vi "MTest.vi"() -> ()   [LabVIEW 2017]
panel:
  in  "Clear W":bool
  out "error out 2":errorcluster
  out "read":string
  in  "Send Cmd":bool
  in  "sendStr":string
  out "RS-232":bool
  in  "Disconnect Com":bool
  in  "Connect Com":bool
  out "TesterVersion":string
  out "error out":errorcluster
  in  "9":bool
  in  "8":bool
  in  "7":bool
  in  "6":bool
  in  "1":bool
  in  "5":bool
  in  "4":bool
  in  "3":bool
  in  "2":bool
  out "DAQ":bool
  in  "Disconnect DAQ":bool
  in  "Connect DAQ":bool
  in  "Stop Button":bool
  in  "Remote":bool
  in  "UP":bool
  in  "DOWN":bool
  in  "V En":bool
  in  "FW":bool
  # "REDLER TECHNOLOGIES LTD"
  # "M Kinetics Tester"
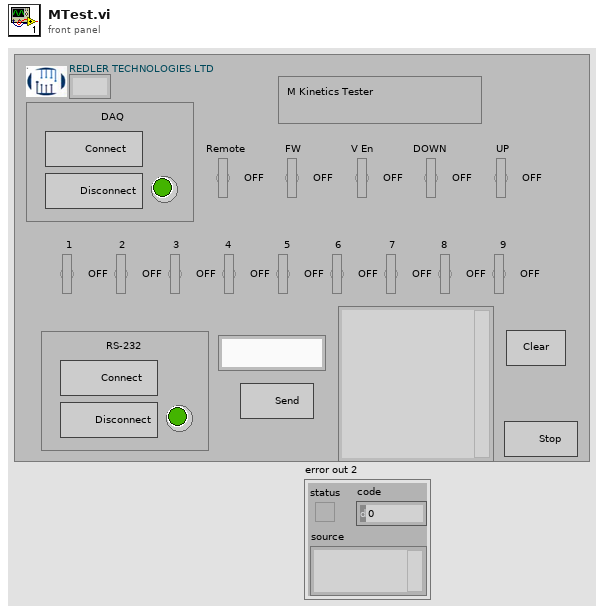
[diagram p1: front panel]
types:
  T1 = enum16{"Init", "0 ohm", "6 ohm", "13.2 ohm", "15 ohm", "25.9 ohm", "33 ohm", "Down", "Up", "Venable", "Firmware", "PowerSuply"}
  T2 = enum16{"Init", "0 ohm", "6 ohm", "13.2 ohm", "15 ohm", "25.9 ohm", "33 ohm", "Down", "Up", "Venable", "Firmware", "PowerSuply"}[]
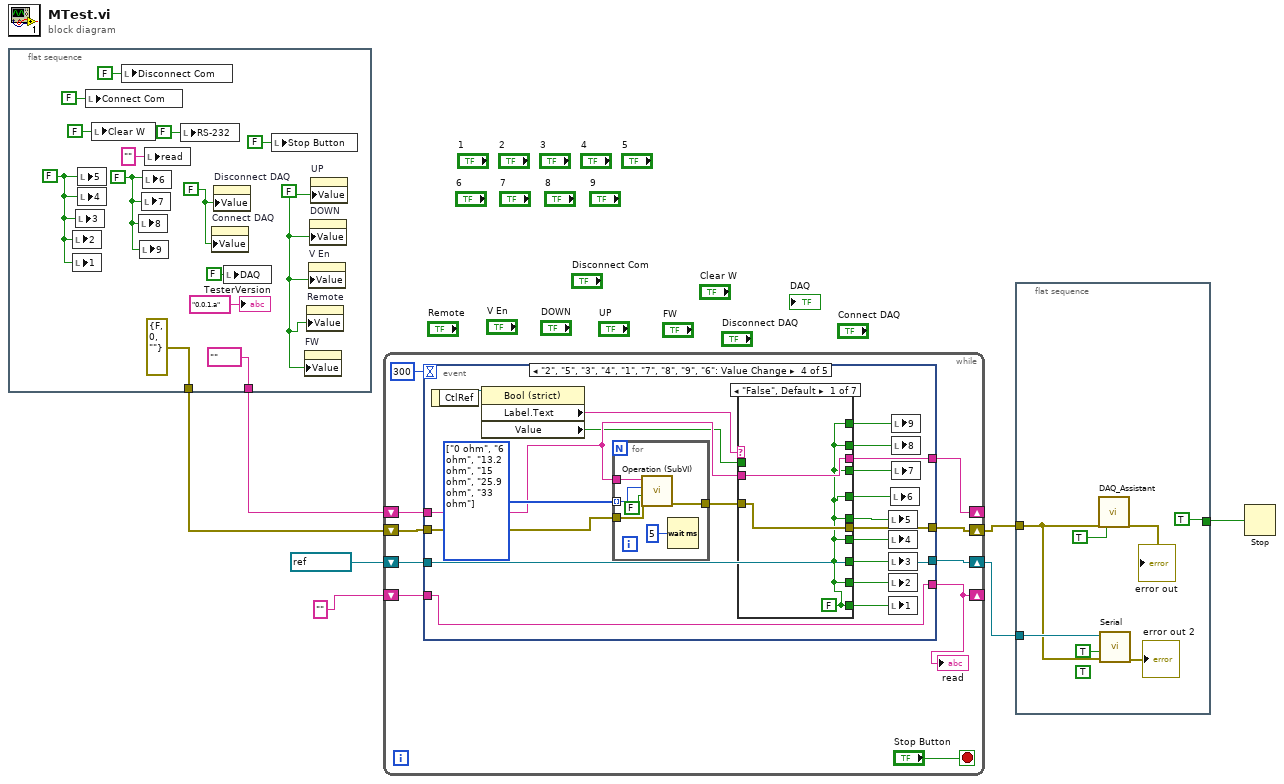
[diagram p0: block diagram]
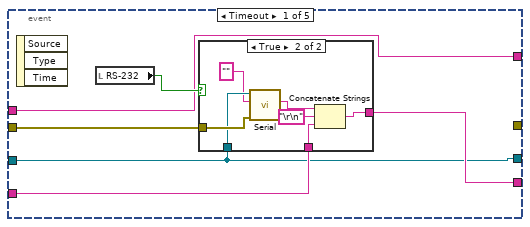
[diagram p2: hidden frame]
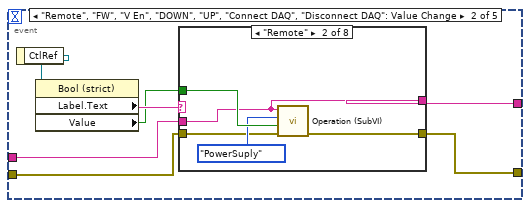
[diagram p4: hidden frame]
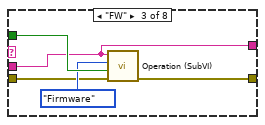
[diagram p6: hidden frame]
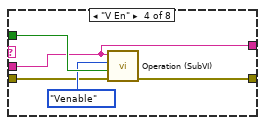
[diagram p7: hidden frame]
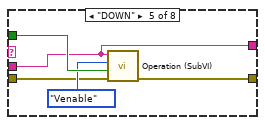
[diagram p8: hidden frame]
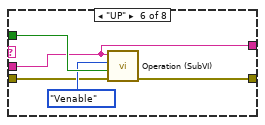
[diagram p9: hidden frame]
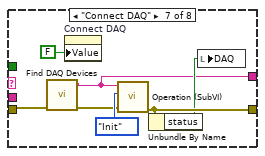
[diagram p10: hidden frame]
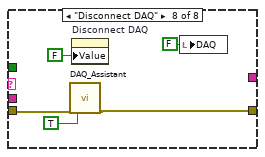
[diagram p11: hidden frame]
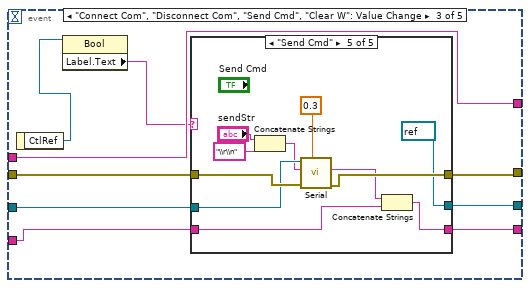
[diagram p12: hidden frame]
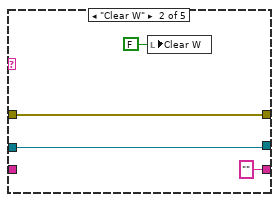
[diagram p14: hidden frame]
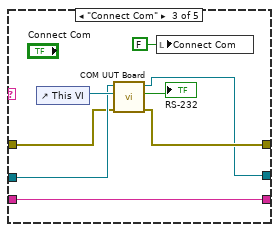
[diagram p15: hidden frame]
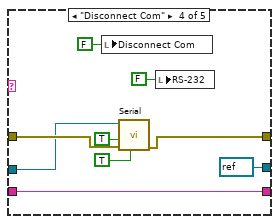
[diagram p16: hidden frame]
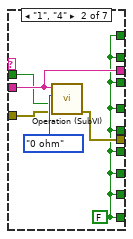
[diagram p17: hidden frame]
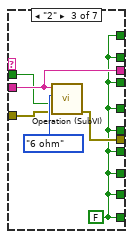
[diagram p18: hidden frame]
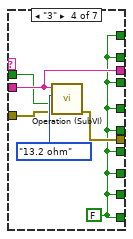
[diagram p19: hidden frame]
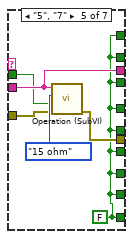
[diagram p20: hidden frame]
diagram:
  n1 = flat-sequence {
    tunnel: [errorcluster {"status"=FALSE, "code"=0, "source"=""} ("error out")] -> w7
    tunnel: [tag "" ("DAQmx Device Name")] -> w6
    frame #0 {
      w15 = FALSE ("6")
      w14 = FALSE ("5")
      w19 = FALSE ("Stop Button")
      w21 = FALSE ("UP")
      n2 = local write "2"(w14) -> ()
      n3 = local write "1"(w14) -> ()
      n4 = local write "3"(w14) -> ()
      n5 = local write "5"(w14) -> ()
      n6 = local write "4"(w14) -> ()
      n7 = local write "Connect Com"(FALSE ("Connect Com")) -> ()
      n8 = local write "Clear W"(FALSE ("Clear W")) -> ()
      n9 = local write "Disconnect Com"(FALSE ("Disconnect Com")) -> ()
      n10 = local write "8"(w15) -> ()
      n11 = local write "9"(w15) -> ()
      n12 = local write "7"(w15) -> ()
      n13 = local write "6"(w15) -> ()
      n14 = local write "read"("" ("read")) -> ()
      n15 = local write "RS-232"(FALSE ("RS-232")) -> ()
      n16 = property on="Connect DAQ" class="Bool (strict)"("Value"=w19) -> ()  [unwired: 2 in, 2 out]
      n17 = property on="Disconnect DAQ" class="Bool (strict)"("Value"=w19) -> ()  [unwired: 2 in, 2 out]
      n18 = local write "DAQ"(FALSE ("DAQ")) -> ()
      n19 = local write "Stop Button"(FALSE ("Stop Button")) -> ()
      n20 = property on="FW" class="Bool (strict)"("Value"=w21) -> ()  [unwired: 2 in, 2 out]
      n21 = property on="Remote" class="Bool (strict)"("Value"=w21) -> ()  [unwired: 2 in, 2 out]
      n22 = property on="V En" class="Bool (strict)"("Value"=w21) -> ()  [unwired: 2 in, 2 out]
      n23 = property on="DOWN" class="Bool (strict)"("Value"=w21) -> ()  [unwired: 2 in, 2 out]
      n24 = property on="UP" class="Bool (strict)"("Value"=w21) -> ()  [unwired: 2 in, 2 out]
      "TesterVersion" <- "0.0.1.a" ("TesterVersion")
    }
  }
  n25 = while {
    shift-right: [w29] -> w5
    shift-left: w7 -> [w30]
    shift-right: [w28] -> _
    shift-left: w6 -> [w31]
    shift-right: [w25] -> w2
    shift-left: refnum<visa-resource-name> "COMx" ("VISA Kinetics") -> [w26]
    shift-right: [w23] -> _
    shift-left: "" -> [w24]
    stop <- "Stop Button" stop-if-true
    n26 = event shown="[3] \"2\", \"5\", \"3\", \"4\", \"1\", \"7\", \"8\", \"9\", \"6\": Value Change" {
      selector: _ -> [_ _ _ _ _]
      dyn-events: _ -> [_ _ _ _ _]
      timeout: 300 -> [_ _ _ _ _]
      tunnel: w31 -> [w34 w50 w98 w151 w206]
      tunnel: w30 -> [w33 w49 w99 w154 w204]
      tunnel: [_ w48 w97 w149 w203] -> w29
      tunnel: [w34 w47 w98 w148 w206] -> w28
      tunnel: w26 -> [w32 _ w95 w136 w201]
      tunnel: [w32 _ w94 w136 w201] -> w25
      tunnel: w24 -> [w36 _ w93 w137 w202]
      tunnel: [w35 _ w92 w137 w202] -> w23
      event Timeout {
        n27 = event-data() -> ()  [unwired: 1 in, 3 out]
        n28 = local read "RS-232"() -> (w37:bool)
        n29 = case shown="True" w37 {
          tunnel: w36 -> [w38 w41]
          tunnel: [w38 w45] -> w35
          tunnel: w33 -> [_ w44]
          tunnel: w32 -> [_ w43]
          frame False {
          }
          frame True {
            n30 = call "Serial.vi"("error in (no error)"=w44, "write buffer"="", "VISA resource name"=w43) -> ("read buffer"=w42:string)  [unwired: 7 in, 1 out]
            n31 = Concatenate Strings(w42, "\r\n", w41) -> (w45:string)
          }
        }
      }
      event "Remote", "FW", "V En", "DOWN", "UP", "Connect DAQ", "Disconnect DAQ": Value Change {
        n32 = event-data() -> ("CtlRef"=w52:refnum<vi>)  [unwired: 1 in]
        n33 = property class="Bool (strict)"(reference=w52) -> ("Label.Text"=w51:string, "Value"=w46:bool)  [unwired: 1 in, 2 out]
        n34 = case shown="\"Remote\"" w51 {
          tunnel: w50 -> [w54 w55 w60 w65 w70 w75 _ _]
          tunnel: w46 -> [_ w59 w64 w69 w74 w79 _ _]
          tunnel: [w53 w57 w62 w67 w72 w77 w84 w89] -> w48
          tunnel: w49 -> [w53 w56 w61 w66 w71 w76 w82 w91]
          tunnel: [w54 w55 w60 w65 w70 w75 w80 _] -> w47
          frame "False", Default {
          }
          frame "Remote" {
            n35 = call "Operation (SubVI).vi"("error in (no error)"=w56, "On/Off"=w59, "Operation"=T1."PowerSuply", "DAQmx Device Name"=w55) -> ("error out"=w57:errorcluster)  [unwired: 7 in]
          }
          frame "FW" {
            n36 = call "Operation (SubVI).vi"("error in (no error)"=w61, "On/Off"=w64, "Operation"=T1."Firmware", "DAQmx Device Name"=w60) -> ("error out"=w62:errorcluster)  [unwired: 7 in]
          }
          frame "V En" {
            n37 = call "Operation (SubVI).vi"("error in (no error)"=w66, "On/Off"=w69, "Operation"=T1."Venable", "DAQmx Device Name"=w65) -> ("error out"=w67:errorcluster)  [unwired: 7 in]
          }
          frame "DOWN" {
            n38 = call "Operation (SubVI).vi"("error in (no error)"=w71, "On/Off"=w74, "Operation"=T1."Venable", "DAQmx Device Name"=w70) -> ("error out"=w72:errorcluster)  [unwired: 7 in]
          }
          frame "UP" {
            n39 = call "Operation (SubVI).vi"("error in (no error)"=w76, "On/Off"=w79, "Operation"=T1."Venable", "DAQmx Device Name"=w75) -> ("error out"=w77:errorcluster)  [unwired: 7 in]
          }
          frame "Connect DAQ" {
            n40 = call "Find DAQ Devices.vi"("Error In"=w82) -> ("Error Out"=w81:errorcluster, "DAQmx Device Name"=w80:tag)  [unwired: 8 in, 1 out]
            n41 = property on="Connect DAQ" class="Bool (strict)"("Value"=FALSE ("Connect DAQ")) -> ()  [unwired: 2 in, 2 out]
            n42 = call "Operation (SubVI).vi"("error in (no error)"=w81, "Operation"=T1."Init", "DAQmx Device Name"=w80) -> ("error out"=w84:errorcluster)  [unwired: 8 in]
            n43 = Unbundle By Name(w84) -> ("status"=w83:bool)
            n44 = local write "DAQ"(w83) -> ()
          }
          frame "Disconnect DAQ" {
            n45 = call "DAQ_Assistant.vi"("error in"=w91, "stop (T)"=TRUE) -> ("error out"=w89:errorcluster)  [unwired: 16 in, 1 out]
            n46 = property on="Disconnect DAQ" class="Bool (strict)"("Value"=FALSE ("Disconnect DAQ")) -> ()  [unwired: 2 in, 2 out]
            n47 = local write "DAQ"(FALSE ("DAQ")) -> ()
          }
        }
      }
      event "Connect Com", "Disconnect Com", "Send Cmd", "Clear W": Value Change {
        n48 = event-data() -> ("CtlRef"=w100:refnum<vi>)  [unwired: 1 in]
        n49 = property class="Bool"(reference=w100) -> ("Label.Text"=w96:string)  [unwired: 1 in, 2 out]
        n50 = case shown="\"Send Cmd\"" w96 {
          tunnel: w99 -> [w102 w106 w112 w124 w135]
          tunnel: [w102 w106 w111 w123 w134] -> w97
          tunnel: w95 -> [w103 w107 w114 w120 w133]
          tunnel: [w103 w107 w110 refnum<visa-resource-name> refnum ("VISA resource name out") refnum<visa-resource-name> refnum ("VISA resource name out")] -> w94
          tunnel: w93 -> [w101 _ w109 w117 w126]
          tunnel: [w101 "" w109 w117 w125] -> w92
          frame "False", Default {
          }
          frame "Clear W" {
            n51 = local write "Clear W"(FALSE ("Clear W")) -> ()
          }
          frame "Connect Com" {
            n52 = control-ref of="This VI"() -> (w115:refnum<vi>)
            n53 = call "COM UUT Board.vi"("error in (no error)"=w112, "VI reference (current VI)"=w115, "VISA resource name 2"=w114) -> ("error out"=w111:errorcluster, ".not. x?"=→"RS-232":bool, "VISA resource name out"=w110:refnum<visa-resource-name>)  [unwired: 6 in]
            n54 = local write "Connect Com"(FALSE ("Connect Com")) -> ()
          }
          frame "Disconnect Com" {
            n55 = local write "Disconnect Com"(FALSE ("Disconnect Com")) -> ()
            n56 = call "Serial.vi"("Close"=TRUE, "error in (no error)"=w124, "Clear Log"=TRUE, "VISA resource name"=w120) -> ("error out"=w123:errorcluster)  [unwired: 6 in, 1 out]
            n57 = local write "RS-232"(FALSE ("RS-232")) -> ()
          }
          frame "Send Cmd" {
            n58 = Concatenate Strings("sendStr", "\\r\\n" ("string")) -> (w129:string)
            n59 = call "Serial.vi"("Delay Time (s)"=0.3, "error in (no error)"=w135, "write buffer"=w129, "VISA resource name"=w133) -> ("error out"=w134:errorcluster, "read buffer"=w127:string)  [unwired: 6 in]
            n60 = Concatenate Strings(w127, w126) -> (w125:string)
          }
        }
      }
      event "2", "5", "3", "4", "1", "7", "8", "9", "6": Value Change {
        w153 = T2 [enum."0 ohm", enum."6 ohm", enum."13.2 ohm", enum."15 ohm", enum."25.9 ohm", enum."33 ohm"] items=["Init", "0 ohm", "6 ohm", "13.2 ohm", "15 ohm", "25.9 ohm", "33 ohm", "Down", "Up", "Venable", "Firmware", "PowerSuply"]
        n61 = event-data() -> ("CtlRef"=w155:refnum<vi>)  [unwired: 1 in]
        n62 = property class="Bool (strict)"(reference=w155) -> ("Label.Text"=w152:string, "Value"=w147:bool)  [unwired: 1 in, 2 out]
        n63 = for {
          tunnel: w153 -> [w199] mode=indexing
          tunnel: w151 -> [w200]
          tunnel: w154 -> [w198]
          tunnel: [w196] -> w150
          n64 = call "Operation (SubVI).vi"("error in (no error)"=w198, "On/Off"=FALSE, "Operation"=w199, "DAQmx Device Name"=w200) -> ("error out"=w196:errorcluster)  [unwired: 7 in]
          n65 = Wait (ms)(milliseconds to wait=u32 5) -> ()  [unwired: 1 out]
        }
        n66 = case shown="\"False\", Default" w152 {
          tunnel: w151 -> [w158 w161 w167 w173 w179 w185 w191]
          tunnel: w150 -> [w157 w163 w169 w175 w181 w187 w193]
          tunnel: [w157 w162 w168 w174 w180 w186 w192] -> w149
          tunnel: [w158 w161 w167 w173 w179 w185 w191] -> w148
          tunnel: w147 -> [_ w160 w166 w172 w178 w184 w190]
          tunnel: [w156 w159 w165 w171 w177 w183 w189] -> w146
          tunnel: [w156 w159 w165 w171 w177 w183 w189] -> w145
          tunnel: [w156 w159 w165 w171 w177 w183 w189] -> w144
          tunnel: [w156 w159 w165 w171 w177 w183 w189] -> w143
          tunnel: [w156 w159 w165 w171 w177 w183 w189] -> w142
          tunnel: [w156 w159 w165 w171 w177 w183 w189] -> w141
          tunnel: [w156 w159 w165 w171 w177 w183 w189] -> w140
          tunnel: [w156 w159 w165 w171 w177 w183 w189] -> w139
          tunnel: [w156 w159 w165 w171 w177 w183 w189] -> w138
          frame "False", Default {
            w156 = FALSE
          }
          frame "1", "4" {
            w159 = FALSE
            n67 = call "Operation (SubVI).vi"("error in (no error)"=w163, "On/Off"=w160, "Operation"=T1."0 ohm", "DAQmx Device Name"=w161) -> ("error out"=w162:errorcluster)  [unwired: 7 in]
          }
          frame "2" {
            w165 = FALSE
            n68 = call "Operation (SubVI).vi"("error in (no error)"=w169, "On/Off"=w166, "Operation"=T1."6 ohm", "DAQmx Device Name"=w167) -> ("error out"=w168:errorcluster)  [unwired: 7 in]
          }
          frame "3" {
            w171 = FALSE
            n69 = call "Operation (SubVI).vi"("error in (no error)"=w175, "On/Off"=w172, "Operation"=T1."13.2 ohm", "DAQmx Device Name"=w173) -> ("error out"=w174:errorcluster)  [unwired: 7 in]
          }
          frame "5", "7" {
            w177 = FALSE
            n70 = call "Operation (SubVI).vi"("error in (no error)"=w181, "On/Off"=w178, "Operation"=T1."15 ohm", "DAQmx Device Name"=w179) -> ("error out"=w180:errorcluster)  [unwired: 7 in]
          }
          frame "6", "9" {
            w183 = FALSE
            n71 = call "Operation (SubVI).vi"("error in (no error)"=w187, "On/Off"=w184, "Operation"=T1."25.9 ohm", "DAQmx Device Name"=w185) -> ("error out"=w186:errorcluster)  [unwired: 7 in]
          }
          frame "8" {
            w189 = FALSE
            n72 = call "Operation (SubVI).vi"("error in (no error)"=w193, "On/Off"=w190, "Operation"=T1."33 ohm", "DAQmx Device Name"=w191) -> ("error out"=w192:errorcluster)  [unwired: 7 in]
          }
        }
        n73 = local write "5"(w141) -> ()
        n74 = local write "4"(w140) -> ()
        n75 = local write "3"(w139) -> ()
        n76 = local write "2"(w138) -> ()
        n77 = local write "1"(w146) -> ()
        n78 = local write "6"(w142) -> ()
        n79 = local write "9"(w145) -> ()
        n80 = local write "8"(w144) -> ()
        n81 = local write "7"(w143) -> ()
      }
      event "Stop Button": Value Change {
        n82 = event-data() -> ()  [unwired: 1 in, 1 out]
        n83 = call "DAQ_Assistant.vi"("error in"=w204, "stop (T)"=TRUE) -> ("error out"=w203:errorcluster)  [unwired: 16 in, 1 out]
      }
    }
    "read" <- w23
  }
  n84 = flat-sequence {
    tunnel: w5 -> [w208]
    tunnel: [TRUE] -> w4
    tunnel: w2 -> [w209]
    frame #0 {
      (unwired) TRUE ("Close")
      n85 = call "DAQ_Assistant.vi"("error in"=w208, "stop (T)"=TRUE) -> ("error out"=→"error out":errorcluster)  [unwired: 16 in, 1 out]
      n86 = call "Serial.vi"("error in (no error)"=w208, "Clear Log"=TRUE, "VISA resource name"=w209) -> ("error out"=→"error out 2":errorcluster)  [unwired: 7 in, 1 out]
    }
  }
  n87 = Stop(stop? (T)=w4) -> ()
